vi "RampsLogicSystem1.vi"() -> ()   [LabVIEW 2017]
panel:
  in  "stage2Clear?":bool
  in  "button2Pushed?":bool
  in  "buttonPushed?":bool
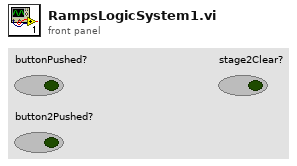
[diagram p1: front panel]
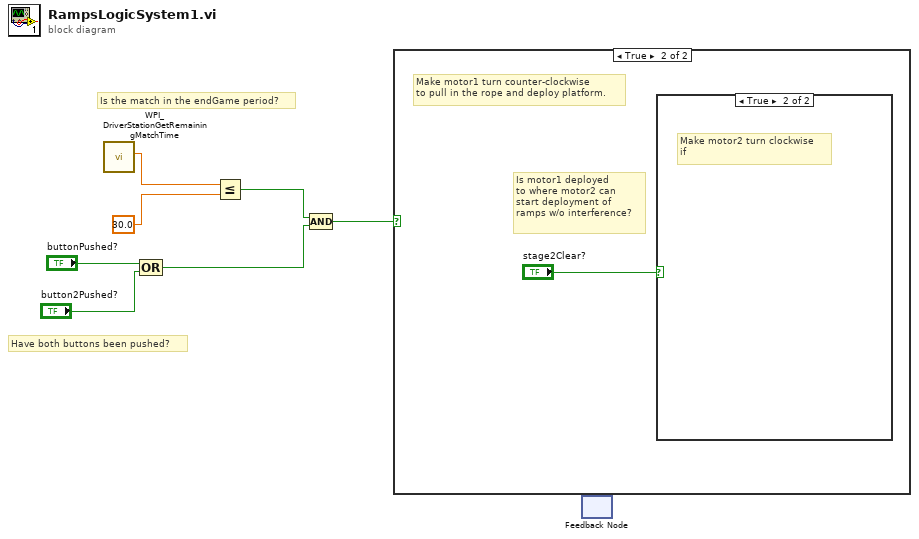
[diagram p0: block diagram]
diagram:
  # "Have both buttons been pushed?"
  # "Is the match in the endGame period?"
  n1 = call <vilib>:"WPI_DriverStationGetRemainingMatchTime.vi"() -> ("Match Time(s)"=w7:sgl)  [unwired: 10 in, 1 out]
  n2 = Compound Arithmetic op=OR("buttonPushed?", "button2Pushed?") -> (w2:bool)
  n3 = Less Or Equal?(x=w7, y=sgl 30.0 ("Match Time(s)")) -> (x <= y?=w5:bool)
  n4 = Compound Arithmetic op=AND(w5, w2) -> (w1:bool)
  n5 = case shown="True" w1 {
    frame False {
    }
    frame True {
      # "Is motor1 deployed\nto where motor2 can\nstart deployment of \nramps w/o interference?"
      # "Make motor1 turn counter-clockwise\nto pull in the rope and deploy platform."
      n6 = case shown="True" "stage2Clear?" {
        frame False {
        }
        frame True {
          # "Make motor2 turn clockwise\nif"
        }
      }
    }
  }
  n7 = feedback-in #1() -> ()  [unwired: 1 out]
  n8 = feedback #1() -> ()  [unwired: 2 in]
